vi "Async Tree Load.vi"(8 "error in (no error)":errorcluster, 11 "QControlWizard in":refnum<class "QControl Creation Wizard.lvclass">) -> (3 "QControlWizard (dup)":refnum<class "QControl Creation Wizard.lvclass">)   [LabVIEW 2020, in "QControl Creation Wizard.lvclass"]
uses:
  QControl Creation Wizard.lvclass
  QControl Classes/TreeControl/Tree Action Enum.ctl
  QControl Classes/TreeControl/Add Item Info Cluster.ctl
  QControl Creation Wizard.lvclass/QControl Creation Wizard.ctl
  QControl Classes/TreeSelectionSingle/TreeSelectionSingle.lvclass
  C:/ODP/QControlToolkit/QControl Classes/TreeControl/TreeControl.lvclass
  C:/ODP/QControlToolkit/QControl Classes/Control/Control.lvclass
  C:/ODP/QControlToolkit/QControl Classes/TreeSelection/TreeSelection.lvclass
  QControl Classes/TreeControl/TreeControl.lvclass
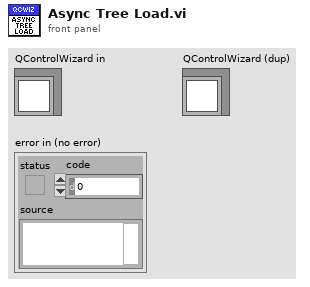
[diagram p1: front panel]
types:
  T1 = typedef "TreeControl.lvclass/Add Item Info Cluster.ctl" = cluster{"Parent Tag (\"\")":string, "Child Position (-1=End)":i32, "Left Cell String (\"\" = Same as Child Tag)":string, "Child Text[]":string[], "Child Tag":string, "Child Only? (F)":bool}
  T2 = typedef "TreeControl.lvclass/Tree Action Enum.ctl" = enum16{"Open All", "Close All", "Open Item", "Close Item"}
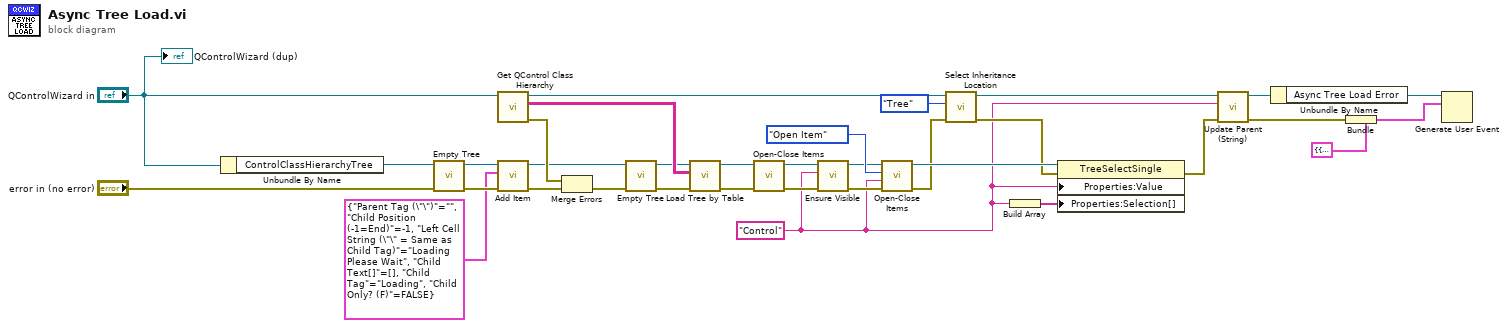
[diagram p0: block diagram]
diagram:
  w16 = "Control" ("Tag (\"\")")
  n1 = Unbundle By Name("QControlWizard in") -> ("ControlClassHierarchyTree"=w34:refnum<class "TreeSelectionSingle.lvclass">)
  n2 = call "Empty Tree.vi"("error in (no error)"="error in (no error)", "Tree in"=w34) -> ("error out"=w14:errorcluster, "Tree (dup)"=w15:refnum<class "TreeSelectionSingle.lvclass">)  [unwired: 8 in]
  n3 = call "Get QControl Class Hierarchy.vi"("ControlClassWizard in"="QControlWizard in") -> ("error out"=w11:errorcluster, "QControl Class Hierarchy"=w19:string[][], "ControlClassWizard out"=w20:refnum<class "QControl Creation Wizard.lvclass">)  [unwired: 8 in]
  n4 = call-dynamic "Add Item.vi"("error in (no error)"=w14, "ItemInfo"=T1 {"Parent Tag (\"\")"="", "Child Position (-1=End)"=-1, "Left Cell String (\"\" = Same as Child Tag)"="Loading Please Wait", "Child Text[]"=[], "Child Tag"="Loading", "Child Only? (F)"=FALSE}, "Tree in"=w15) -> ("error out"=w13:errorcluster, "Tree out"=w10:refnum<class "TreeSelectionSingle.lvclass">)  [unwired: 6 in, 1 out]
  n5 = Merge Errors(w11, w13) -> (w9:errorcluster)
  n6 = call "Empty Tree.vi"("error in (no error)"=w9, "Tree in"=w10) -> ("error out"=w7:errorcluster, "Tree (dup)"=w8:refnum<class "TreeSelectionSingle.lvclass">)  [unwired: 8 in]
  n7 = call-dynamic "Load Tree by Table.vi"("error in (no error)"=w7, "Table"=w19, "Tree in"=w8) -> ("error out"=w27:errorcluster, "Tree out"=w28:refnum<class "TreeSelectionSingle.lvclass">)  [unwired: 7 in]
  n8 = call-dynamic "Open-Close Items.vi"("error in (no error)"=w27, "Tree in"=w28) -> ("error out"=w25:errorcluster, "Tree (dup)"=w26:refnum<class "TreeSelectionSingle.lvclass">)  [unwired: 8 in]
  n9 = call "Ensure Visible.vi"("error in (no error)"=w25, "Tag"=w16, "Tree in"=w26) -> ("error out"=w29:errorcluster, "Tree out"=w30:refnum<class "TreeSelectionSingle.lvclass">)  [unwired: 7 in]
  n10 = call-dynamic "Open-Close Items.vi"("error in (no error)"=w29, "Tag (\"\")"=w16, "Action (Close All)"=Tree_Action_Enum."Open Item", "Tree in"=w30) -> ("error out"=w23:errorcluster, "Tree (dup)"=w32:refnum<class "TreeSelectionSingle.lvclass">)  [unwired: 6 in]
  n11 = call "Select Inheritance Location.vi"("error in (no error)"=w23, "NewVal"=enum32{"Tree", "Path"}."Tree", "QControlWizard in"=w20) -> ("error out"=w22:errorcluster, "QControlWizard (dup)"=w18:refnum<class "QControl Creation Wizard.lvclass">)  [unwired: 7 in]
  n12 = Build Array(w16) -> (w33:string[])
  n13 = property class="TreeSelectSingle"(reference=w32, error in=w22, "Properties:Value"=w16, "Properties:Selection[]"=w33) -> (error out=w17:errorcluster)  [unwired: 1 out]
  n14 = call "Update Parent (String).vi"("error in (no error)"=w17, "Parent Name"=w16, "ControlClassWizard in"=w18) -> ("error out"=w4:errorcluster, "ControlClassWizard (dup)"=w6:refnum<class "QControl Creation Wizard.lvclass">)  [unwired: 7 in]
  n15 = Unbundle By Name(w6) -> ("Async Tree Load Error"=w5:refnum<user-event>)
  n16 = Bundle(cluster=cluster{"error?":errorcluster} {"error?"={"status"=FALSE, "code"=0, "source"=""}}, "error?"=w4) -> (w3:cluster{"error?":errorcluster})
  n17 = Generate User Event(user event=w5, event data cluster=w3) -> ()  [unwired: 2 in, 2 out]
  "QControlWizard (dup)" <- "QControlWizard in"
